vi "ReadFreqVoltage.vi"(8 "error in (no error)":errorcluster, 11 "channel":tag="Dev1/ai1") -> (0 "error out":errorcluster, 2 "Ampl":dbl, 3 "frequency":dbl format="%.2p", 4 "Waveform":dbl[](array[numeric]), 5 "Avg":dbl format="%.2p")   [LabVIEW 2011]
uses:
  <vilib>/DAQmx/read.llb/DAQmx Read (Analog Wfm 1Chan NSamp).vi
  <vilib>/DAQmx/create/channels.llb/DAQmx Create Channel (AI-Voltage-Basic).vi
  <vilib>/DAQmx/configure/timing.llb/DAQmx Timing (Sample Clock).vi
  <vilib>/measure/matone.llb/Extract Single Tone Information 1 Chan.vi
  <vilib>/DAQmx/miscellaneous.llb/DAQmx Fill In Error Info.vi
  <vilib>/measure/NI_MAPro.lvlib
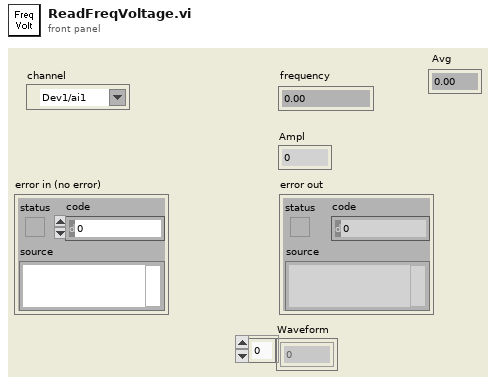
[diagram p1: front panel]
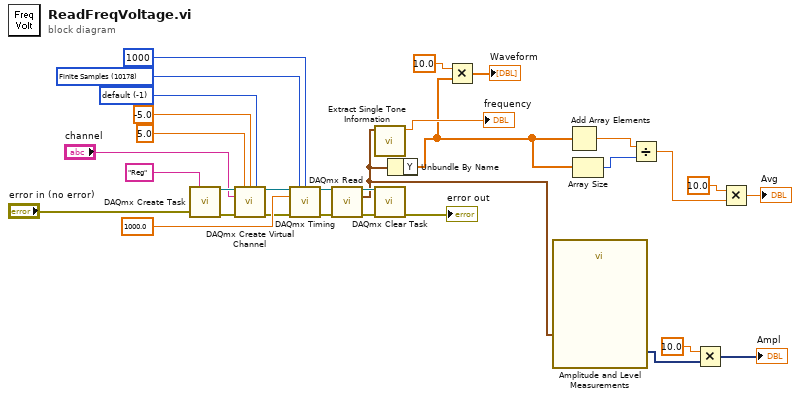
[diagram p0: block diagram]
diagram:
  w26 = -1 items=["default"=-1, "RSE"=10083, "NRSE"=10078, "Differential"=10106, "Pseudodifferential"=12529] ("config")
  w23 = 10178 items=["Finite Samples"=10178, "Continuous Samples"=10123, "Hardware Timed Single Point"=12522] ("sample mode")
  n1 = call <vilib>:"DAQmx Create Task.vi"("new task name"="Reg", "error in"="error in (no error)") -> ("task out"=w30:refnum<k21>, "error out"=w25:errorcluster)  [unwired: 3 in, 9 out]
  n2 = call-poly <vilib>:"DAQmx Create Virtual Channel.vi"("task in"=w30, "maximum value"=5.0, "minimum value"=-5.0, "input terminal configuration"=w26, "physical channels"="channel", "error in"=w25) -> ("task out"=w24:refnum<k21>, "error out"=w21:errorcluster)  [unwired: 3 in, 5 out]
  n3 = call-poly <vilib>:"DAQmx Timing.vi"("task/channels in"=w24, "sample mode"=w23, "samples per channel"=1000 ("smpperch"), "rate"=1000.0, "error in"=w21) -> ("task out"=w18:refnum<k21>, "error out"=w16:errorcluster)  [unwired: 2 in, 7 out]
  n4 = call-poly <vilib>:"DAQmx Read.vi"("task/channels in"=w18, "error in"=w16) -> ("task out"=w17:refnum<k21>, "data"=w9:waveform(dbl), "error out"=w15:errorcluster)  [unwired: 1 in, 10 out]
  n5 = call-poly <vilib>:"Extract Single Tone Information.vi"("time signal in"=w9) -> ("detected frequency"=→"frequency":dbl)  [unwired: 3 in, 7 out]
  n6 = call <vilib>:"DAQmx Clear Task.vi"("task in"=w17, "error in"=w15) -> ("error out"=→"error out":errorcluster)  [unwired: 13 out]
  n7 = Unbundle By Name(w9) -> ("Y"=w2:dbl[])
  n8 = Multiply(x=10.0 ("y"), y=w2) -> (x*y=→"Waveform":dbl[])
  n9 = call "Amplitude and Level Measurements"("Signals"=w9) -> ("Positive Peak"=w10:dynamicdata)  [unwired: 1 in, 13 out]
  n10 = Add Array Elements(numeric array=w2) -> (sum=w8:dbl)
  n11 = Array Size(array=w2) -> (size(s)=w7:i32)
  n12 = Divide(x=w8, y=w7) -> (x/y=w5:dbl)
  n13 = Multiply(x=10.0 ("y"), y=w10) -> (x*y=→"Ampl":dynamicdata)
  n14 = Multiply(x=10.0 ("y"), y=w5) -> (x*y=→"Avg":dbl)
